vi "Periodic Tasks.vi"(8 "error in":errorcluster) -> ()   [LabVIEW 2017]
doc: "This VI runs in parallel to other tasks. It can contain as many user-defined periodic loops as you need. These can carry out PID or other sorts of timed response."
panel:
  out "Sensor 2":bool
  out "Estado":dbl
  out "Sensor 1":bool
  out "Valor Motor":dbl
  in  "Segurando":dbl
  in  "Expelir":dbl
  in  "Coletar":dbl
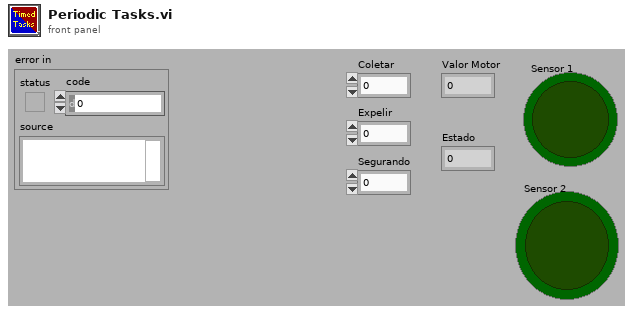
[diagram p1: front panel]
types:
  T1 = enum16{"Repouso", "Coletar", "Segurando", "Expelindo"}
  T2 = typedef "WPI_JoystickDevRef.ctl" = cluster{"Device":T3}
  T3 = typedef "WPI_JoystickDeviceEnum.ctl" = enum16{"USB 0", "USB 1", "USB 2", "USB 3", "USB 4", "USB 5"}
  T4 = typedef "WPI_SwitchDevRef.ctl" = cluster{"DevStatus":errorcluster, "DIO Channel":T5, "CntIndex":T6, "Normally Closed":bool}
  T5 = typedef "FPGA_DIOChannel.ctl" = enum8{"DIO 0", "DIO 1", "DIO 2", "DIO 3", "DIO 4", "DIO 5", "DIO 6", "DIO 7", "DIO 8", "DIO 9", "DIO MXP 0", "DIO MXP 1", "DIO MXP 2", "DIO MXP 3", "DIO MXP 4", "DIO MXP 5", "DIO MXP 6", "DIO MXP 7", "DIO MXP 8", "DIO MXP 9", "DIO MXP 10", "DIO MXP 11", "DIO MXP 12", "DIO MXP 13", "DIO MXP 14", "DIO MXP 15", "SPI Port CS1", "SPI Port CS2", "SPI Port CS3", "SPI Port MISO", "SPI Port MOSI", "Invalid"}
  T6 = typedef "FPGA_CounterCtrSystemIndex.ctl" = enum8{"Ctr 0", "Ctr 1", "Ctr 2", "Ctr 3", "Ctr 4", "Ctr 5", "Ctr 6", "Ctr 7", "Invalid"}
  T7 = cluster{"Buttons[0]":bool, "Buttons[1]":bool, "Buttons[2]":bool, "Buttons[3]":bool, "Buttons[4]":bool, "Buttons[5]":bool, "Buttons[6]":bool, "Buttons[7]":bool, "Buttons[8]":bool}
  T8 = typedef "WPI_MotorControlDeviceRef.ctl" = cluster{"DeviceStatus":errorcluster, "Type":T9, "PWM":cluster{"PWM Channel":T10, "DeadBand":T11}, "CAN":cluster{"Device Number":u8, "SetOutput VI Ref":variant, "GetOutput VI Ref":variant, "Enable VI Ref":variant, "Disable VI Ref":variant, "Data":variant}, "Invert":bool, "DIO PWM":cluster{"PWM \"Enable\" Channel":T10, "DIOChannel":T5, "PWM Rate":dbl}}
  T9 = typedef "WPI_MotorControlType.ctl" = enum16{"PWM", "CAN", "DIO PWM"}
  T10 = typedef "FPGA_DIOPWMChannel.ctl" = enum8{"PWM 0", "PWM 1", "PWM 2", "PWM 3", "PWM 4", "PWM 5", "PWM 6", "PWM 7", "PWM 8", "PWM 9", "PWM MXP 0", "PWM MXP 1", "PWM MXP 2", "PWM MXP 3", "PWM MXP 4", "PWM MXP 5", "PWM MXP 6", "PWM MXP 7", "PWM MXP 8", "PWM MXP 9", "Invalid"}
  T11 = typedef "WPI_PWMDeadband.ctl" = cluster{"Name":string, "maxPositivePwm":i32, "minPositivePwm":i32, "centerPwm":i32, "maxNegativePwm":i32, "minNegativePwm":i32, "angularRange":u16}
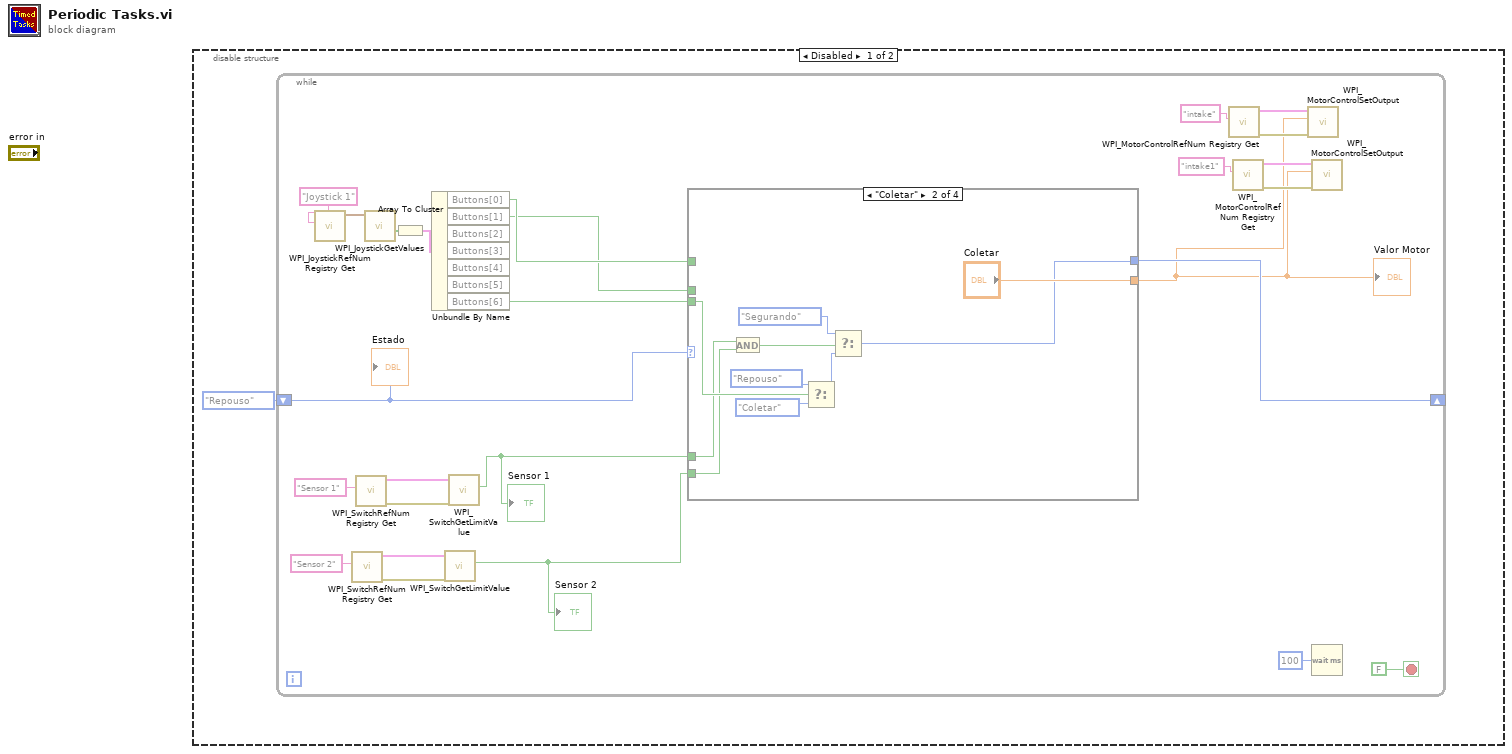
[diagram p0: block diagram]
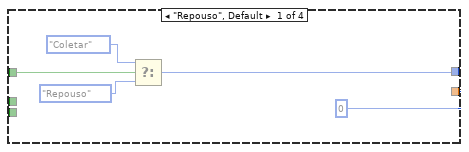
[diagram p2: hidden frame]
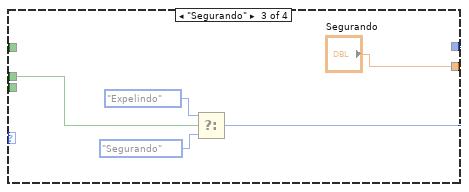
[diagram p3: hidden frame]
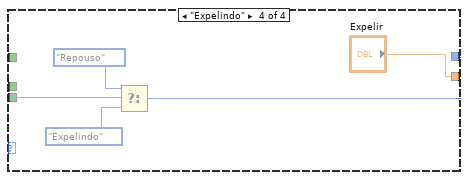
[diagram p4: hidden frame]
diagram:
  n1 = disable-structure shown="Disabled" {
    frame Disabled {
      n2 = while {
        shift-right: [w25] -> _
        shift-left: T1."Repouso" -> [w24]
        stop <- FALSE stop-if-true
        n3 = call <vilib>:"WPI_JoystickRefNum Registry Get.vi"("refnum name"="Joystick 1") -> ("JoystickDevRef"=w10:T2)  [unwired: 1 in, 9 out]
        n4 = call <vilib>:"WPI_SwitchRefNum Registry Get.vi"("refnum name"="Sensor 2") -> ("error out"=w5:errorcluster, "SwitchDevRef"=w4:T4)  [unwired: 9 in]
        n5 = call <vilib>:"WPI_SwitchRefNum Registry Get.vi"("refnum name"="Sensor 1") -> ("error out"=w16:errorcluster, "SwitchDevRef"=w15:T4)  [unwired: 9 in]
        n6 = call <vilib>:"WPI_JoystickGetValues.vi"("JoystickDevRef"=w10) -> ("Buttons"=w11:bool[])  [unwired: 6 in, 4 out]
        n7 = Array To Cluster(array=w11) -> (cluster=w12:T7)
        n8 = Unbundle By Name(w12) -> ("Buttons[0]"=w8:bool, "Buttons[1]"=w7:bool, "Buttons[6]"=w6:bool)  [unwired: 4 out]
        n9 = call <vilib>:"WPI_SwitchGetLimitValue.vi"("error in (no error)"=w5, "SwitchDevRef"=w4) -> ("Switch Pressed"=w2:bool)  [unwired: 7 in, 2 out]
        "Sensor 2" <- w2
        n10 = call <vilib>:"WPI_SwitchGetLimitValue.vi"("error in (no error)"=w16, "SwitchDevRef"=w15) -> ("Switch Pressed"=w13:bool)  [unwired: 7 in, 2 out]
        "Sensor 1" <- w13
        n11 = case shown="\"Coletar\"" w24 {
          tunnel: w8 -> [w31 _ _ _]
          tunnel: [w29 w36 w43 w50] -> w25
          tunnel: [0 "Coletar" "Segurando" "Expelir"] -> w19
          tunnel: w7 -> [_ _ w46 _]
          tunnel: w13 -> [_ w35 _ _]
          tunnel: w6 -> [_ w39 _ w48]
          tunnel: w2 -> [_ w34 _ _]
          frame "Repouso", Default {
            n12 = Select(t=T1."Coletar", s=w31, f=T1."Repouso") -> (s? t:f=w29:T1)
          }
          frame "Coletar" {
            n13 = And(x=w35, y=w34) -> (x .and. y?=w33:bool)
            n14 = Select(t=T1."Repouso", s=w39, f=T1."Coletar") -> (s? t:f=w37:T1)
            n15 = Select(t=T1."Segurando", s=w33, f=w37) -> (s? t:f=w36:T1)
          }
          frame "Segurando" {
            n16 = Select(t=T1."Expelindo", s=w46, f=T1."Segurando") -> (s? t:f=w43:T1)
          }
          frame "Expelindo" {
            n17 = Select(t=T1."Repouso", s=w48, f=T1."Expelindo") -> (s? t:f=w50:T1)
          }
        }
        "Valor Motor" <- w19
        n18 = call <vilib>:"WPI_MotorControlRefNum Registry Get.vi"("refnum name"="intake") -> ("error out"=w21:errorcluster, "MotorControlDevRef"=w20:T8)  [unwired: 9 in]
        n19 = call <vilib>:"WPI_MotorControlRefNum Registry Get.vi"("refnum name"="intake1") -> ("error out"=w23:errorcluster, "MotorControlDevRef"=w22:T8)  [unwired: 9 in]
        n20 = call <vilib>:"WPI_MotorControlSetOutput.vi"("error in (no error)"=w21, "Output"=w19, "MotorControlDevRef"=w20) -> ()  [unwired: 6 in, 3 out]
        n21 = call <vilib>:"WPI_MotorControlSetOutput.vi"("error in (no error)"=w23, "Output"=w19, "MotorControlDevRef"=w22) -> ()  [unwired: 6 in, 3 out]
        n22 = Wait (ms)(milliseconds to wait=u32 100) -> ()  [unwired: 1 out]
        "Estado" <- w24
      }
    }
    frame Enabled {
    }
  }
